vi "Get_T_AVS.vi"(4 "error in (no error)":errorcluster caption="Fehler (Eingang, kein Fehler)", 5 "AVS-Channel":dbl, 6 "AVS-Excitation":dbl, 7 "AVS-VISA":refnum<visa-resource-name>) -> (0 "error out":errorcluster caption="Fehler (Ausgang)", 1 "Resistance reading":dbl format="%.2f", 2 "T (K)":dbl=0.00957168277075326 format="%^.3e", 3 "dup AVS-VISA":refnum<visa-resource-name>)   [LabVIEW 2019]
uses:
  Instrument_Setup.vi
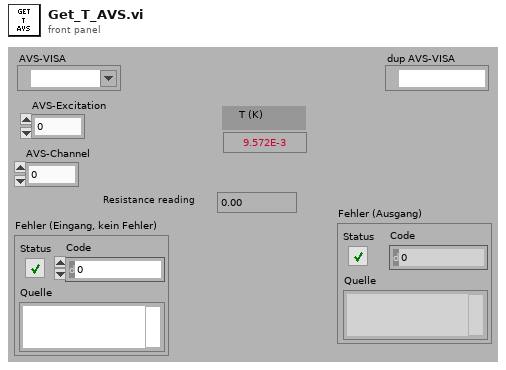
[diagram p1: front panel]
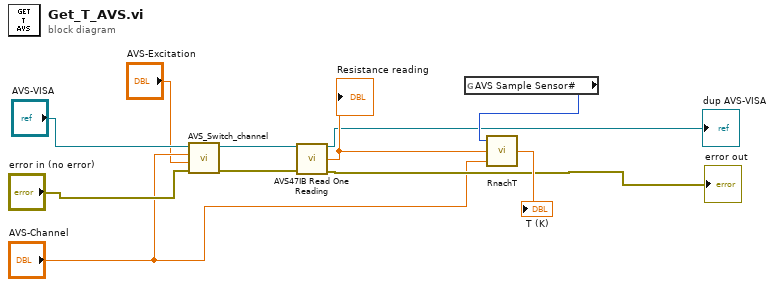
[diagram p0: block diagram]
diagram:
  n1 = call "AVS_Switch_channel.vi"("error in (no error) 3"="error in (no error)", "AVS Excitation"="AVS-Excitation", "AVS Channel"="AVS-Channel", "AVS-VISA"="AVS-VISA") -> ("error out (no error) 2"=w3:errorcluster, "dup VISA-AVS"=w4:refnum<visa-resource-name>)  [unwired: 6 in]
  n2 = call "AVS47IB Read One Reading.vi"("VISA session"=w4, "error in (no error)"=w3) -> ("dup VISA session"=→"dup AVS-VISA":refnum<visa-resource-name>, "Resistance reading"=w10:dbl, "error out"=→"error out":errorcluster)  [unwired: 9 in, 2 out]
  "Resistance reading" <- w10
  n3 = global read "Instrument_Setup.vi" "AVS Sample Sensor#"() -> (w9:u16)
  n4 = call "RnachT.vi"("AVS Channel"="AVS-Channel", "R"=w10, "Sensor Cal#"=w9) -> ("T (K)"=→"T (K)":dbl)
